vi "SelfParking_Final.vi"() -> ()   [LabVIEW 2020]
uses:
  <vilib>/Instr/_visa.llb/VISA Flush IO Buffer Mask.ctl
  <vilib>/Instr/_visa.llb/VISA Configure Serial Port (Instr).vi
panel:
  out "Intruder Alert":bool
  out "Access Granted":bool
  out "Done":bool
  out "Parallel":bool
  out "Perpendicular":bool
  out "Output String":string
  in  "Module Path":path
  in  "Stop 2":bool
  out "Centimeters":i32
  in  "Stop1":bool
  out "Parallel":bool
  out "Perpendicular":bool
  out "Scanning":bool
  out "Ask user":bool
  out "Wait for start":bool
  out "Move to stop line":bool
  out "Execute":bool
  in  "VISA resource name":refnum<visa-resource-name>
  # "Voice Access Indicators"
  # "Outputs"
  # "Parking Process & Parking Type Indicators"
  # "Inputs"
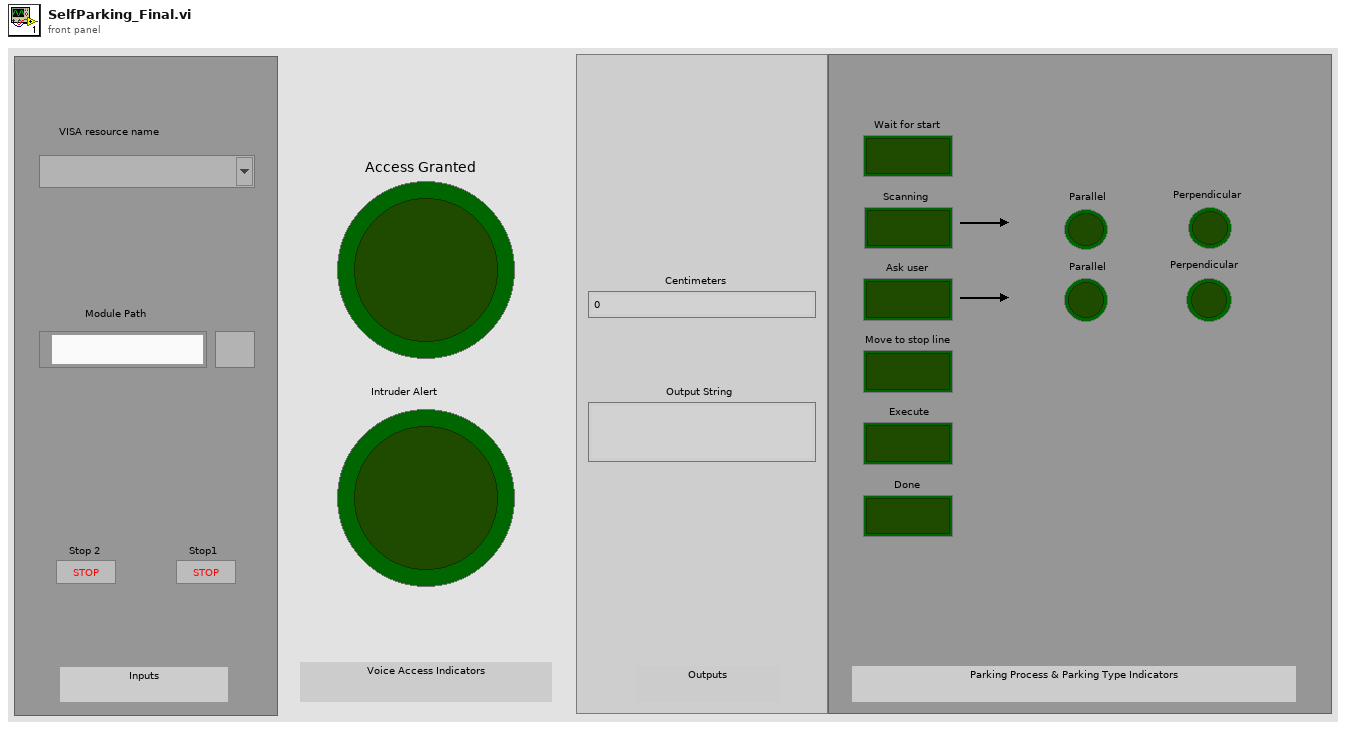
[diagram p1: front panel]
types:
  T1 = enum16{"wait for start", "move to stop line", "scanning", "ask user", "execute park"}
  T2 = enum16{"wait for start", "move to stop line", "scanning", "ask user", "execute park", "Done"}
  T3 = typedef "VISA Flush IO Buffer Mask.ctl" = u16
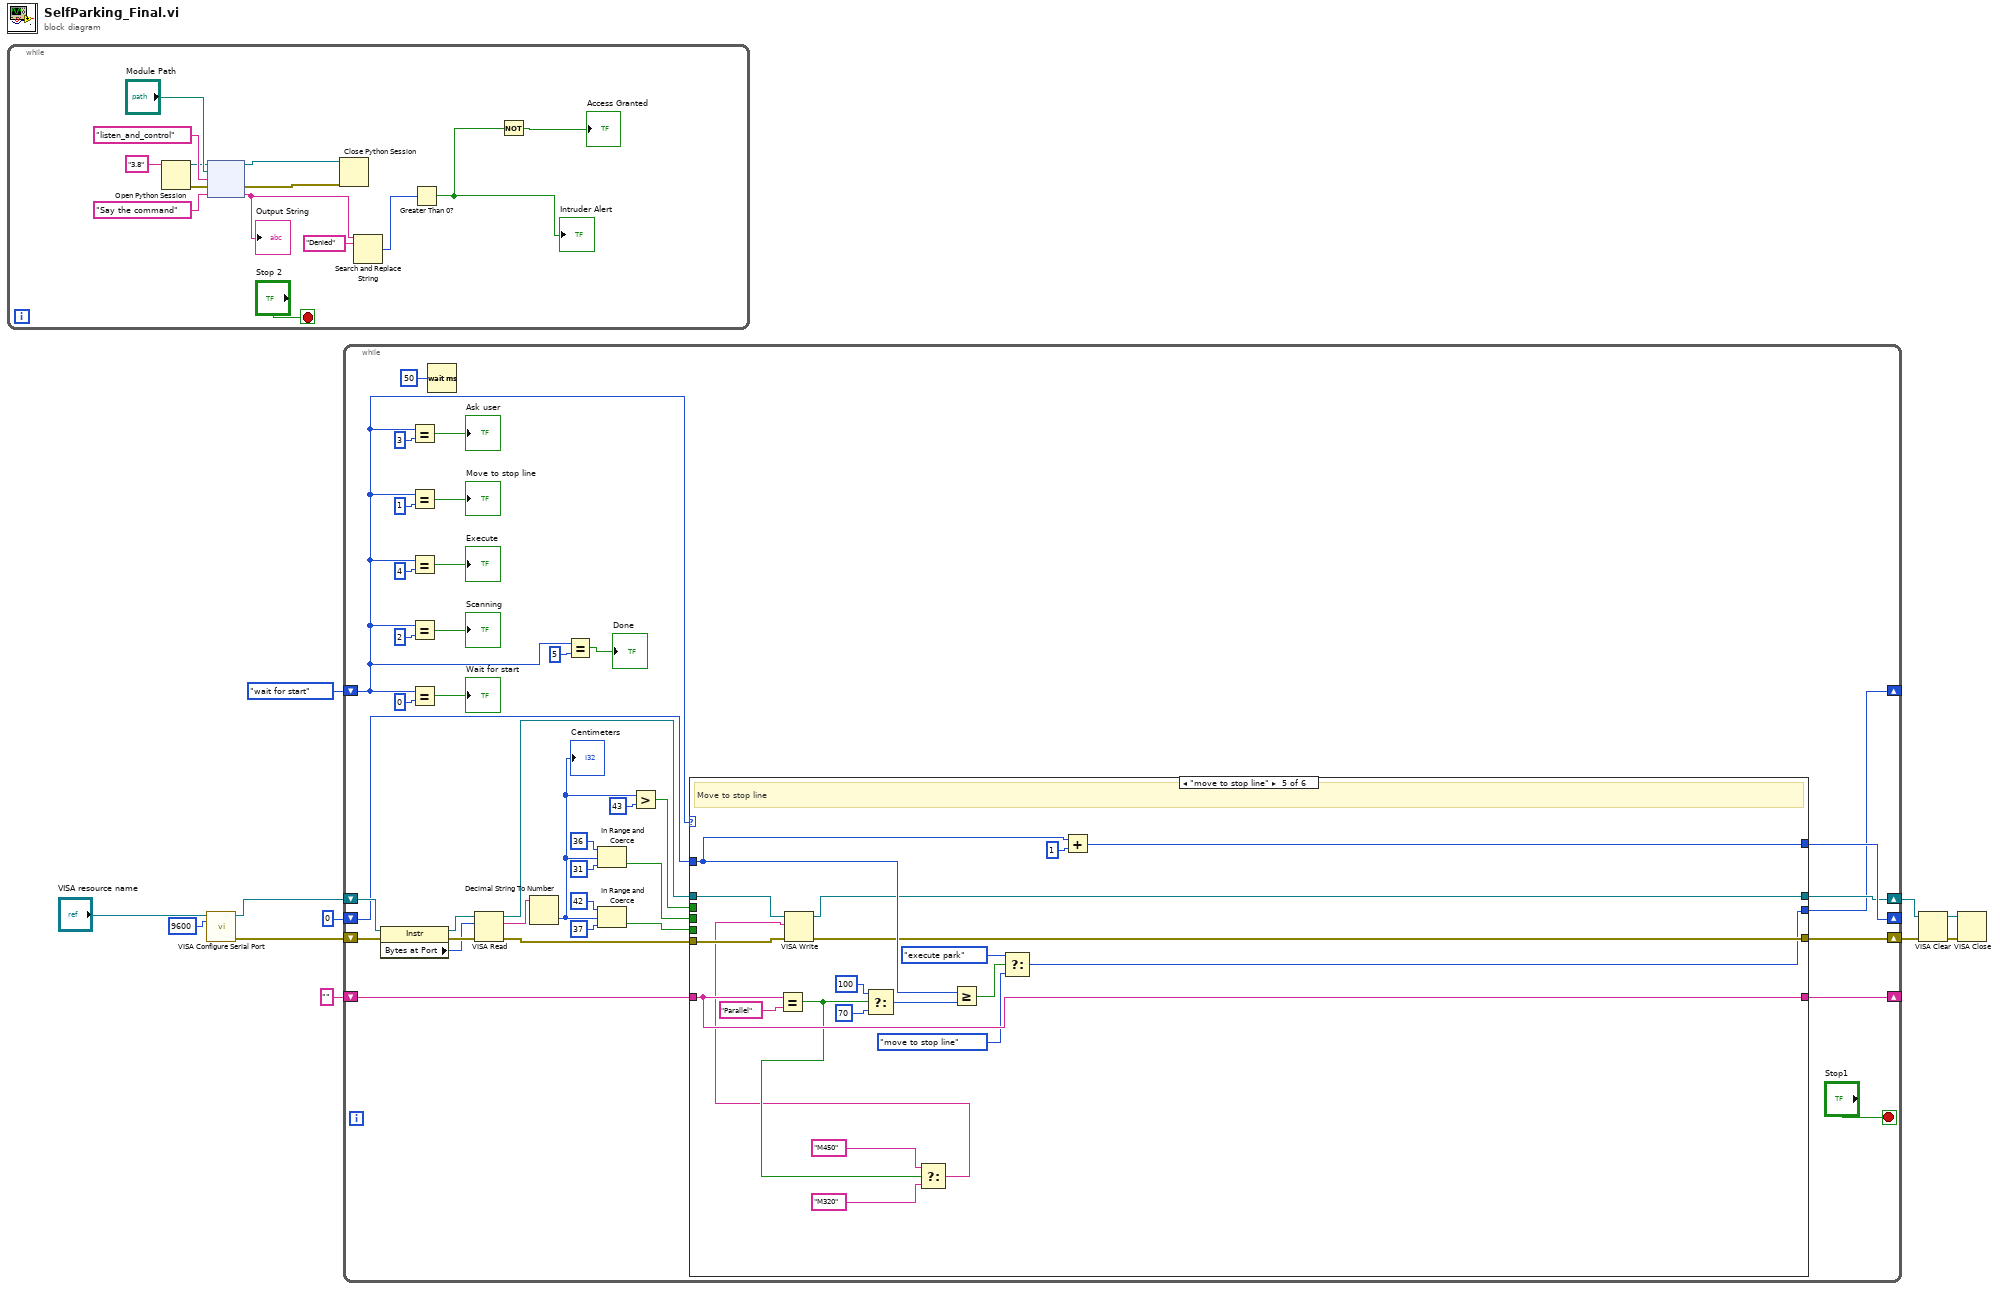
[diagram p0: block diagram]
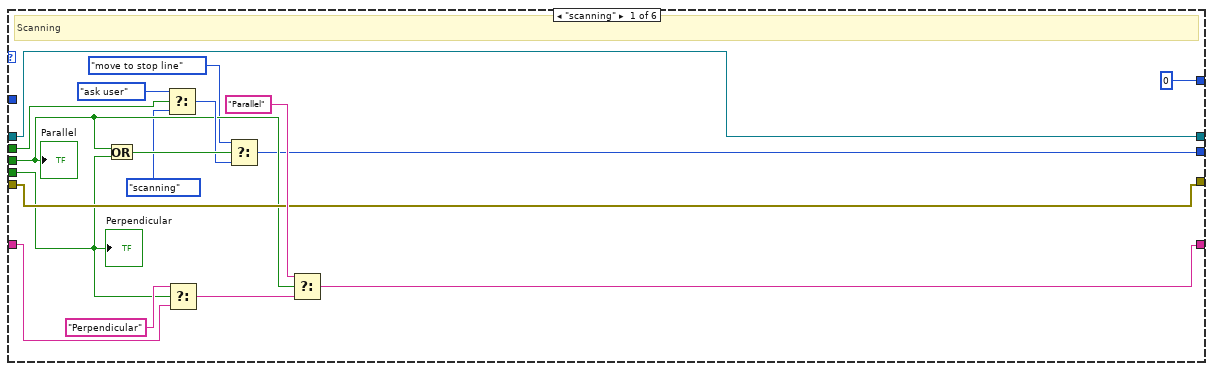
[diagram p2: hidden frame]
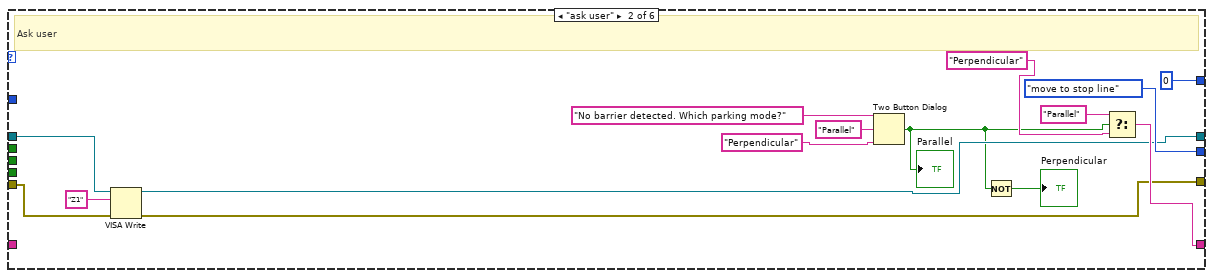
[diagram p3: hidden frame]
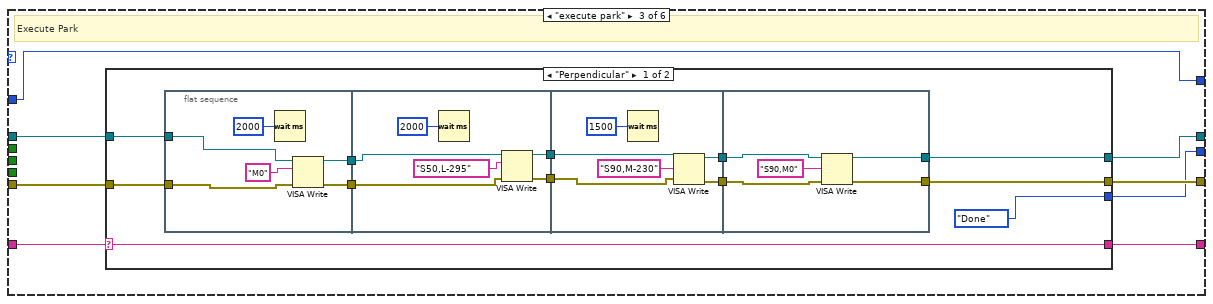
[diagram p4: hidden frame]
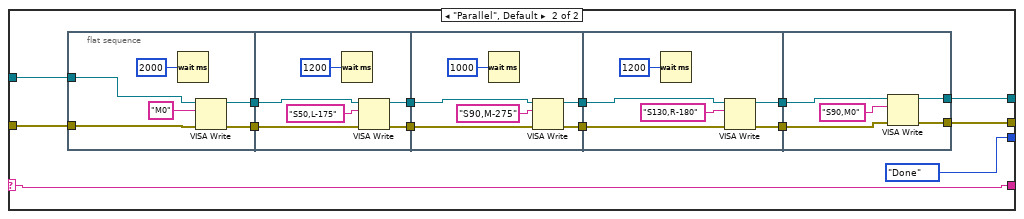
[diagram p5: hidden frame]
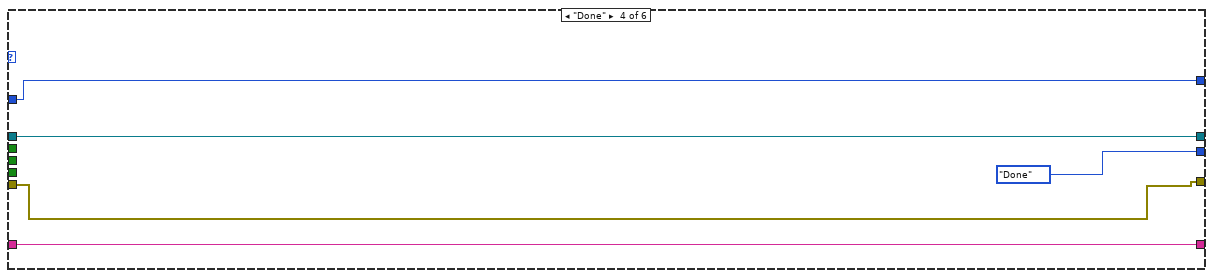
[diagram p6: hidden frame]
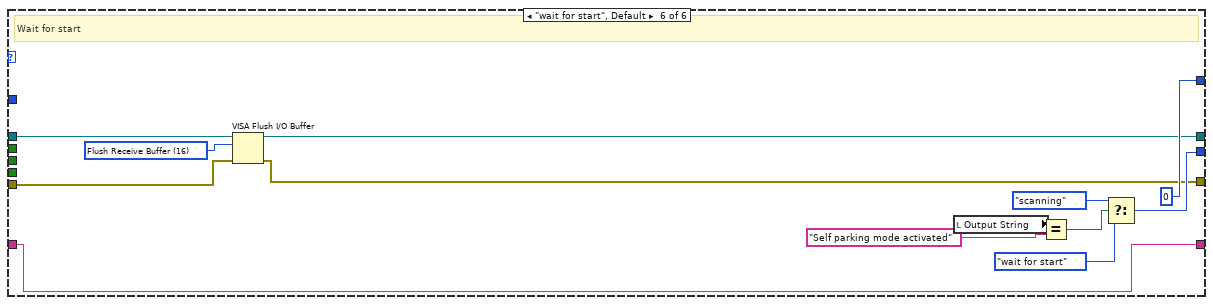
[diagram p7: hidden frame]
diagram:
  n1 = while {
    stop <- "Stop 2" stop-if-true
    n2 = Open Python Session(python version="3.8" ("Python version")) -> (session out=w22:refnum<k35>, error out=w21:errorcluster)  [unwired: 2 in]
    n3 = node(w22, "Module Path", "listen_and_control" ("function name"), w21, "Say the command") -> (w17:refnum<k35>, w20:errorcluster, w16:string)  [unwired: 2 out]
    "Output String" <- w16
    n4 = Close Python Session(session in=w17, error in=w20) -> ()  [unwired: 1 out]
    n5 = Search and Replace String(input string=w16, search string="Denied") -> (number of replacements=w14:i32)  [unwired: 6 in, 3 out]
    n6 = Greater Than 0?(x=w14) -> (x > 0?=w12:bool)
    "Intruder Alert" <- w12
    n7 = Not(x=w12) -> (.not. x?=→"Access Granted":bool)
  }
  n8 = call-poly "VISA Configure Serial Port"("VISA resource name"="VISA resource name", "baud rate (9600)"=u32 9600) -> ("VISA resource name out"=w9:refnum<visa-resource-name>, "error out"=w8:errorcluster)  [unwired: 12 in]
  n9 = while {
    shift-right: [w48] -> w4
    shift-left: w9 -> [w61]
    shift-right: [w47] -> w2
    shift-left: w8 -> [w59]
    shift-right: [w54] -> _
    shift-left: 0 -> [w53]
    shift-right: [w51] -> _
    shift-left: "" -> [w52]
    shift-right: [w29] -> _
    shift-left: T1."wait for start" -> [w26]
    stop <- "Stop1" stop-if-true
    n10 = property class="Instr"(reference=w61, error in=w59) -> (reference out=w60:refnum<visa-resource-name>, error out=w58:errorcluster, "Bytes at Port"=w57:u32)
    n11 = Equal?(x=w26, y=u16 3) -> (x = y?=→"Ask user":bool)
    n12 = Equal?(x=w26, y=u16 1) -> (x = y?=→"Move to stop line":bool)
    n13 = Equal?(x=w26, y=u16 4) -> (x = y?=→"Execute":bool)
    n14 = Equal?(x=w26, y=u16 2) -> (x = y?=→"Scanning":bool)
    n15 = Equal?(x=w26, y=u16 0) -> (x = y?=→"Wait for start":bool)
    n16 = Wait (ms)(milliseconds to wait=u32 50) -> ()  [unwired: 1 out]
    n17 = VISA Read(VISA resource name=w60, byte count=w57, error in (no error)=w58) -> (VISA resource name out=w49:refnum<visa-resource-name>, read buffer=w64:string, error out=w46:errorcluster)  [unwired: 1 out]
    n18 = Decimal String To Number(string=w64) -> (number=w30:i32)  [unwired: 2 in, 1 out]
    "Centimeters" <- w30
    n19 = Equal?(x=w26, y=u16 5) -> (x = y?=→"Done":bool)
    n20 = In Range and Coerce(upper limit=36, x=w30, lower limit=31) -> (In Range?=w56:bool)  [unwired: 1 out]
    n21 = In Range and Coerce(upper limit=42, x=w30, lower limit=37) -> (In Range?=w55:bool)  [unwired: 1 out]
    n22 = Greater?(x=w30, y=43) -> (0:w50:bool)
    n23 = case shown="\"move to stop line\"" w26 {
      tunnel: w56 -> [w71 _ _ _ _ _]
      tunnel: w55 -> [w70 _ _ _ _ _]
      tunnel: [0 0 w103 w184 w201 0] -> w54
      tunnel: w53 -> [_ _ w103 w184 w203 _]
      tunnel: w52 -> [w78 _ w104 w187 w207 w220]
      tunnel: [w76 w91 w98 w187 w207 w220] -> w51
      tunnel: w50 -> [w69 _ _ _ _ _]
      tunnel: w49 -> [w74 w88 w102 w186 w200 w212]
      tunnel: w46 -> [w73 w87 w101 w183 w199 w210]
      tunnel: [w74 w85 w100 w186 w198 w211] -> w48
      tunnel: [w73 w84 w99 w183 w197 w209] -> w47
      tunnel: [w68 T1."move to stop line" w97 T2."Done" w196 w213] -> w29
      frame "scanning" {
        # "Scanning"
        n24 = Or(x=w71, y=w70) -> (x .or. y?=w79:bool)
        n25 = Select(t=T1."ask user", s=w69, f=T1."scanning") -> (s? t:f=w75:T1)
        n26 = Select(t="Perpendicular", s=w70, f=w78) -> (s? t:f=w77:string)
        n27 = Select(t=T1."move to stop line", s=w79, f=w75) -> (s? t:f=w68:T1)
        n28 = Select(t="Parallel", s=w71, f=w77) -> (s? t:f=w76:string)
        "Parallel" <- w71
        "Perpendicular" <- w70
      }
      frame "ask user" {
        # "Ask user"
        n29 = VISA Write(VISA resource name=w88, write buffer="Z1", error in (no error)=w87) -> (VISA resource name out=w85:refnum<visa-resource-name>, error out=w84:errorcluster)  [unwired: 1 out]
        n30 = Two Button Dialog(message="No barrier detected. Which parking mode?", 1:"Perpendicular" ("F button name (\"Cancel\")"), 2:"Parallel" ("T button name (\"OK\")")) -> (T button?=w83:bool)
        "Parallel" <- w83
        n31 = Not(x=w83) -> (.not. x?=→"Perpendicular":bool)
        n32 = Select(t="Parallel", s=w83, f="Perpendicular") -> (s? t:f=w91:string)
      }
      frame "execute park" {
        # "Execute Park"
        n33 = case shown="\"Perpendicular\"" w104 {
          selector: w104 -> [w116 w153]
          tunnel: [w116 w153] -> w98
          tunnel: w102 -> [w115 w143]
          tunnel: w101 -> [w114 w142]
          tunnel: [T2."Done" T2."Done"] -> w97
          tunnel: [w109 w146] -> w100
          tunnel: [w108 w145] -> w99
          frame "Perpendicular" {
            n34 = flat-sequence {
              tunnel: w114 -> [w122]
              tunnel: w115 -> [w119]
              tunnel: [w121] -> w107
              tunnel: [w120] -> w106
              tunnel: [w126] -> w113
              tunnel: [w125] -> w112
              tunnel: w107 -> [w124]
              tunnel: w106 -> [w123]
              tunnel: w113 -> [w132]
              tunnel: w112 -> [w131]
              tunnel: [w130] -> w111
              tunnel: [w129] -> w110
              tunnel: w111 -> [w138]
              tunnel: w110 -> [w137]
              tunnel: [w136] -> w109
              tunnel: [w135] -> w108
              frame #0 {
                n35 = Wait (ms)(milliseconds to wait=u32 2000) -> ()  [unwired: 1 out]
                n36 = VISA Write(VISA resource name=w119, write buffer="M0", error in (no error)=w122) -> (VISA resource name out=w121:refnum<visa-resource-name>, error out=w120:errorcluster)  [unwired: 1 out]
              }
              frame #1 {
                n37 = Wait (ms)(milliseconds to wait=u32 2000) -> ()  [unwired: 1 out]
                n38 = VISA Write(VISA resource name=w124, write buffer="S50,L-295", error in (no error)=w123) -> (VISA resource name out=w126:refnum<visa-resource-name>, error out=w125:errorcluster)  [unwired: 1 out]
              }
              frame #2 {
                n39 = Wait (ms)(milliseconds to wait=u32 1500) -> ()  [unwired: 1 out]
                n40 = VISA Write(VISA resource name=w132, write buffer="S90,M-230", error in (no error)=w131) -> (VISA resource name out=w130:refnum<visa-resource-name>, error out=w129:errorcluster)  [unwired: 1 out]
              }
              frame #3 {
                n41 = VISA Write(VISA resource name=w138, write buffer="S90,M0", error in (no error)=w137) -> (VISA resource name out=w136:refnum<visa-resource-name>, error out=w135:errorcluster)  [unwired: 1 out]
              }
            }
          }
          frame "Parallel", Default {
            n42 = flat-sequence {
              tunnel: w143 -> [w157]
              tunnel: w142 -> [w156]
              tunnel: [w155] -> w141
              tunnel: [w154] -> w140
              tunnel: [w163] -> w152
              tunnel: [w162] -> w149
              tunnel: w141 -> [w161]
              tunnel: w140 -> [w160]
              tunnel: w152 -> [w169]
              tunnel: [w168] -> w151
              tunnel: w149 -> [w167]
              tunnel: [w166] -> w148
              tunnel: w151 -> [w175]
              tunnel: [w174] -> w150
              tunnel: w148 -> [w173]
              tunnel: [w172] -> w147
              tunnel: w150 -> [w181]
              tunnel: w147 -> [w180]
              tunnel: [w179] -> w146
              tunnel: [w178] -> w145
              frame #0 {
                n43 = Wait (ms)(milliseconds to wait=u32 2000) -> ()  [unwired: 1 out]
                n44 = VISA Write(VISA resource name=w157, write buffer="M0", error in (no error)=w156) -> (VISA resource name out=w155:refnum<visa-resource-name>, error out=w154:errorcluster)  [unwired: 1 out]
              }
              frame #1 {
                n45 = Wait (ms)(milliseconds to wait=u32 1200) -> ()  [unwired: 1 out]
                n46 = VISA Write(VISA resource name=w161, write buffer="S50,L-175", error in (no error)=w160) -> (VISA resource name out=w163:refnum<visa-resource-name>, error out=w162:errorcluster)  [unwired: 1 out]
              }
              frame #2 {
                n47 = Wait (ms)(milliseconds to wait=u32 1000) -> ()  [unwired: 1 out]
                n48 = VISA Write(VISA resource name=w169, write buffer="S90,M-275", error in (no error)=w167) -> (VISA resource name out=w168:refnum<visa-resource-name>, error out=w166:errorcluster)  [unwired: 1 out]
              }
              frame #3 {
                n49 = Wait (ms)(milliseconds to wait=u32 1200) -> ()  [unwired: 1 out]
                n50 = VISA Write(VISA resource name=w175, write buffer="S130,R-180", error in (no error)=w173) -> (VISA resource name out=w174:refnum<visa-resource-name>, error out=w172:errorcluster)  [unwired: 1 out]
              }
              frame #4 {
                n51 = VISA Write(VISA resource name=w181, write buffer="S90,M0", error in (no error)=w180) -> (VISA resource name out=w179:refnum<visa-resource-name>, error out=w178:errorcluster)  [unwired: 1 out]
              }
            }
          }
        }
      }
      frame "Done" {
      }
      frame "move to stop line" {
        # "Move to stop line"
        n52 = Equal?(x=w207, y="Parallel") -> (x = y?=w189:bool)
        n53 = Select(t=100, s=w189, f=70) -> (s? t:f=w205:i32)
        n54 = Select(t="M450" ("write buffer"), s=w189, f="M320" ("write buffer")) -> (s? t:f=w188:string)
        n55 = VISA Write(VISA resource name=w200, write buffer=w188, error in (no error)=w199) -> (VISA resource name out=w198:refnum<visa-resource-name>, error out=w197:errorcluster)  [unwired: 1 out]
        n56 = Greater Or Equal?(x=w203, y=w205) -> (x >= y?=w204:bool)
        n57 = Select(t=T1."execute park", s=w204, f=T1."move to stop line") -> (s? t:f=w196:T1)
        n58 = Add(x=w203, y=1) -> (x+y=w201:i32)
      }
      frame "wait for start", Default {
        w208 = T3 16 items=["Flush Receive Buffer"=16, "Write Transmit Buffer to Device"=32, "Flush Receive Buffer (No I/O)"=64, "Flush Transmit Buffer"=128] ("Mask")
        # "Wait for start"
        n59 = VISA Flush I/O Buffer(VISA resource name=w212, mask (16)=w208, error in (no error)=w210) -> (VISA resource name out=w211:refnum<visa-resource-name>, error out=w209:errorcluster)
        n60 = local read "Output String"() -> (w215:string)
        n61 = Equal?(x=w215, y="Self parking mode activated") -> (x = y?=w214:bool)
        n62 = Select(t=T1."scanning", s=w214, f=T1."wait for start") -> (s? t:f=w213:T1)
      }
    }
  }
  n63 = VISA Clear(VISA resource name=w4, error in (no error)=w2) -> (VISA resource name out=w3:refnum<visa-resource-name>, error out=w1:errorcluster)
  n64 = VISA Close(VISA resource name=w3, error in (no error)=w1) -> ()  [unwired: 1 out]
